vi "Get Open Projects.vi"(8 "error in (no error)":errorcluster) -> (0 "error out":errorcluster, 2 "Project Names":string[](array[string]), 3 "Project Data":T1[](array[typedef]))   [LabVIEW 2018, in "Covers-o-meter.lvlib"]
uses:
  Covers-o-meter.lvlib
  ctl/Project--cluster.ctl
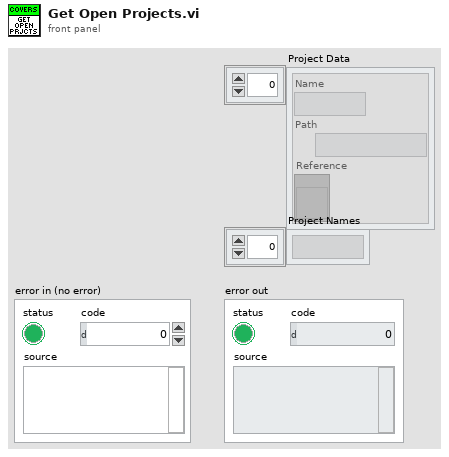
[diagram p1: front panel]
types:
  T1 = typedef "Covers-o-meter.lvlib/Project--cluster.ctl" = cluster{"Name":string, "Path":path, "Reference":refnum<vi>}
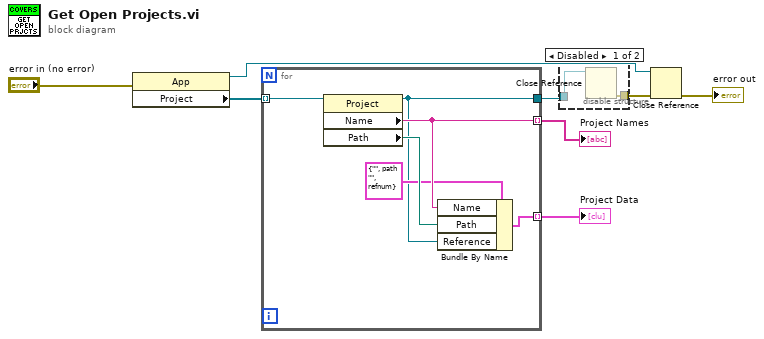
[diagram p0: block diagram]
diagram:
  n1 = property class="App"(error in="error in (no error)") -> (reference out=w5:refnum<vi>, "Project"=w3:refnum<vi>[])  [unwired: 1 in, 1 out]
  n2 = for {
    tunnel: w3 -> [w14] mode=indexing
    tunnel: [w9] -> w4
    tunnel: [w13] -> w2 mode=indexing
    tunnel: [w10] -> w1 mode=indexing
    n3 = property class="Project"(reference=w14) -> (reference out=w9:refnum<vi>, "Name"=w13:string, "Path"=w12:path)  [unwired: 1 in, 1 out]
    n4 = Bundle By Name(cluster=T1 {"Name"="", "Path"=path "", "Reference"=refnum} ("Project"), "Name"=w13, "Path"=w12, "Reference"=w9) -> (w10:T1)
  }
  "Project Data" <- w1
  "Project Names" <- w2
  n5 = disable-structure shown="Disabled" {
    disable-tunnel: [w16 _] -> w6
    disable-tunnel: w4 -> [w15 _]
    frame Disabled {
      n6 = Close Reference(reference=w15) -> (error out=w16:errorcluster)  [unwired: 1 in]
    }
    frame Enabled {
    }
  }
  n7 = Close Reference(reference=w5, error in (no error)=w6) -> (error out=→"error out":errorcluster)
